vi "Get Variable.vi"(6 "wait for reply (T)":bool=TRUE, 8 "error in":errorcluster, 9 "Variable":string, 10 "Socket":i32, 11 "Station ID":i32=-1) -> (0 "error out":errorcluster, 1 "timed out?":bool, 2 "Value":variant, 4 "Get value timed out?":bool, 5 "Variable not found?":bool)   [LabVIEW 2025, in "Test Unit.lvlib"]
doc: "_____\nCreated using DQMH Event Scripter 7.0.1.1316."
uses:
  Test Unit.lvlib
  Get Variable Argument--cluster.ctl
  Get Variable (Reply Payload)--cluster.ctl
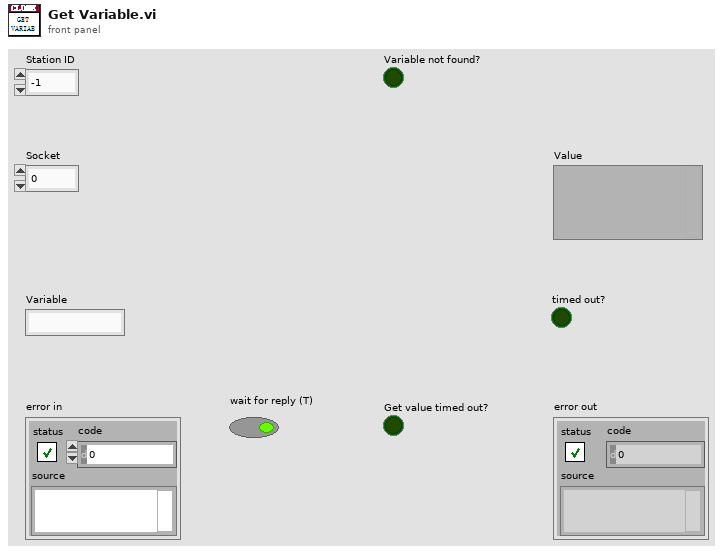
[diagram p1: front panel]
types:
  T1 = typedef "Test Unit.lvlib/Get Variable Argument--cluster.ctl" = cluster{"Module ID":i32, "Socket":i32, "Variable":string, "Wait Notifier":refnum<notifier>, "wait for reply":bool}
  T2 = typedef "Test Unit.lvlib/Request Events--cluster.ctl" = cluster{"Stop Module":refnum<user-event>, "Show Panel":refnum<user-event>, "Hide Panel":refnum<user-event>, "Show Diagram":refnum<user-event>, "Get Module Execution Status":refnum<user-event>, "TileWindows":refnum<user-event>, "TitleWindows":refnum<user-event>, "Cofiguration":refnum<user-event>, "Load Sequence":refnum<user-event>, "Write SN":refnum<user-event>, "UUT Test":refnum<user-event>, "UUTs Test":refnum<user-event>, "Terminate Test":refnum<user-event>, "Set Variable":refnum<user-event>, "Get Variable":refnum<user-event>, "LanguageChanged":refnum<user-event>}
  T3 = typedef "Test Unit.lvlib/Get Variable (Reply Payload)--cluster.ctl" = cluster{"Module ID":i32, "Value":variant, "Variable not found?":bool, "timed out?":bool, "error":errorcluster}
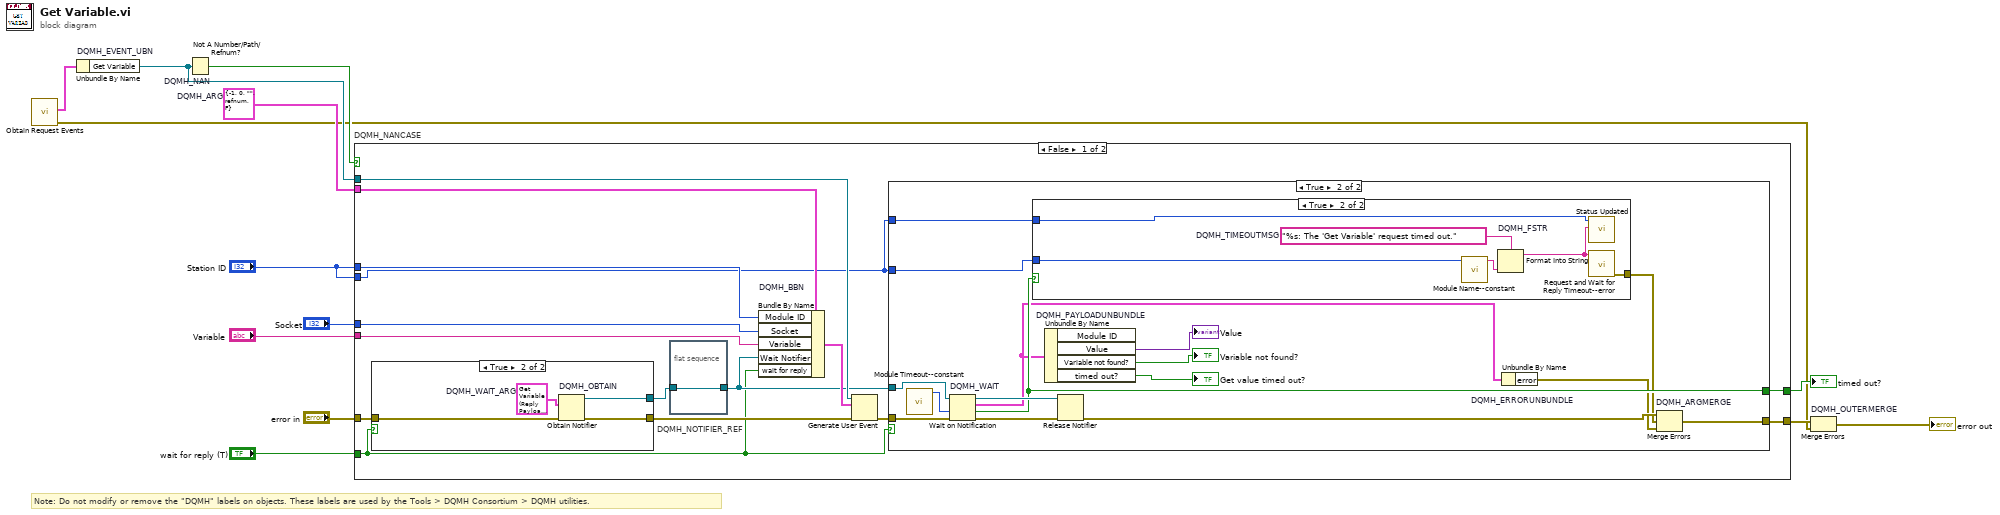
[diagram p0: block diagram]
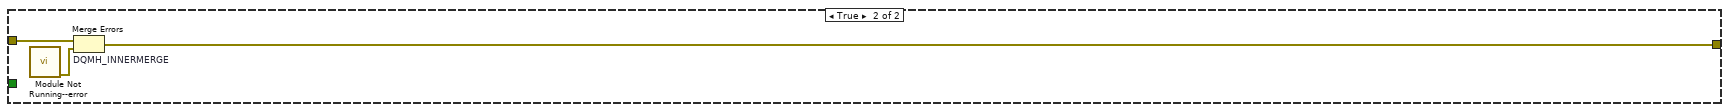
[diagram p5: hidden frame]
diagram:
  w7 = T1 {"Module ID"=-1, "Socket"=0, "Variable"="", "Wait Notifier"=refnum, "wait for reply"=FALSE}  # DQMH_ARG
  # "Note: Do not modify or remove the \"DQMH\" labels on objects. These labels are used by the Tools > DQMH Consortium > DQMH utilities."
  n1 = call "Obtain Request Events.vi"() -> ("error out"=w2:errorcluster, "Test Unit Request Events"=w1:T2)  [unwired: 10 in]
  n2 = Unbundle By Name "DQMH_EVENT_UBN"(w1) -> ("Get Variable"=w11:refnum<user-event>)
  n3 = Not A Number/Path/Refnum? "DQMH_NAN"(number/path/refnum=w11) -> (NaN/Path/Refnum?=w10:bool)
  n4 = case "DQMH_NANCASE" shown="False" w10 {
    tunnel: "error in" -> [w28 w60]
    tunnel: w11 -> [w26 _]
    tunnel: [w23 w59] -> w8
    tunnel: [w24 _] -> w9
    tunnel: w7 -> [w19 _]
    tunnel: "Station ID" -> [w18 _]
    tunnel: "Socket" -> [w17 _]
    tunnel: "Variable" -> [w16 _]
    tunnel: "Station ID" -> [w15 _]
    tunnel: "wait for reply (T)" -> [w14 _]
    frame False {
      n5 = case shown="True" w14 {
        tunnel: w28 -> [w53 w57]
        tunnel: [w53 w56] -> w25
        tunnel: [_ w54] -> w21
        frame False {
        }
        frame True {
          w55 = T3 {"Module ID"=-1, "Value"=variant, "Variable not found?"=FALSE, "timed out?"=FALSE, "error"={"status"=FALSE, "code"=0, "source"=""}}  # DQMH_WAIT_ARG
          n6 = Obtain Notifier "DQMH_OBTAIN"(notification data type=w55, error in (no error)=w57) -> (notifier out=w54:refnum<notifier>, error out=w56:errorcluster)  [unwired: 2 in, 1 out]
        }
      }
      n7 = flat-sequence "DQMH_NOTIFIER_REF" {
        tunnel: w21 -> [w29]
        tunnel: [w29] -> w20
        frame #0 {
        }
      }
      n8 = Bundle By Name "DQMH_BBN"(cluster=w19, "Module ID"=w18, "Socket"=w17, "Variable"=w16, "Wait Notifier"=w20, "wait for reply"=w14) -> (w22:T1)
      n9 = Generate User Event(user event=w26, event data cluster=w22, error in=w25) -> (error out=w27:errorcluster)  [unwired: 1 in, 1 out]
      n10 = case shown="True" w14 {
        tunnel: w27 -> [w30 w46]
        tunnel: w20 -> [_ w45]
        tunnel: [_ w43] -> w24
        tunnel: [w30 w42] -> w23
        tunnel: w15 -> [_ w32]
        tunnel: w15 -> [_ w31]
        frame False {
        }
        frame True {
          n11 = call "Module Timeout--constant.vi"() -> ("Module Timeout"=w36:i32)  [unwired: 11 in]
          n12 = Wait on Notification "DQMH_WAIT"(notifier=w45, timeout in ms (-1)=w36, error in (no error)=w46) -> (notifier out=w44:refnum<notifier>, notification=w37:T3, timed out?=w43:bool, error out=w41:errorcluster)  [unwired: 1 in]
          n13 = case shown="True" w43 {
            tunnel: [_ w50] -> w38
            tunnel: w32 -> [_ w48]
            tunnel: w31 -> [_ w47]
            frame False {
            }
            frame True {
              w52 = "%s: The 'Get Variable' request timed out."  # DQMH_TIMEOUTMSG
              n14 = call "Module Name--constant.vi"("Module ID"=w47) -> ("Module Name"=w49:string)  [unwired: 10 in]
              n15 = Format Into String "DQMH_FSTR"(format string=w52, w49) -> (resulting string=w51:string)  [unwired: 2 in, 1 out]
              n16 = call "Status Updated.vi"("Status"=w51, "Module ID"=w48) -> ()  [unwired: 9 in, 1 out]
              n17 = call "Request and Wait for Reply Timeout--error.vi"("Error Message"=w51) -> ("error out"=w50:errorcluster)  [unwired: 10 in]
            }
          }
          n18 = Unbundle By Name "DQMH_PAYLOADUNBUNDLE"(w37) -> ("Value"=→"Value":variant, "Variable not found?"=→"Variable not found?":bool, "timed out?"=→"Get value timed out?":bool)  [unwired: 1 out]
          n19 = Release Notifier(notifier=w44, error in (no error)=w41) -> (error out=w40:errorcluster)  [unwired: 1 in, 2 out]
          n20 = Unbundle By Name "DQMH_ERRORUNBUNDLE"(w37) -> ("error"=w39:errorcluster)
          n21 = Merge Errors "DQMH_ARGMERGE"(w40, w38, w39) -> (w42:errorcluster)
        }
      }
    }
    frame True {
      n22 = call "Module Not Running--error.vi"() -> ("error out"=w58:errorcluster)  [unwired: 11 in]
      n23 = Merge Errors "DQMH_INNERMERGE"(w60, w58) -> (w59:errorcluster)
    }
  }
  "timed out?" <- w9
  n24 = Merge Errors "DQMH_OUTERMERGE"(w8, w2) -> (→"error out":errorcluster)
